vi "Create Data Channel.vi"(8 "error in (no error)":errorcluster, 9 "Channel":T1 {"Address" format="%.0x"}, 10 "Name":string, 11 "Parent Section":refnum<k24>) -> (0 "error out":errorcluster, 2 "New Data Channel":refnum<k24>, 3 "Parent Section Duplicate":refnum<k24>, 4 "Newly Created?":bool, 6 "Adds Warn?":bool caption="Address Within NIVS Reserved Range?")   [LabVIEW 2010, in "RefMem PtByPt System Definition API.lvlib"]
doc: "Create a data channel to contain the value at the specified reflective memory address."
uses:
  RefMem PtByPt System Definition API.lvlib
  Channel Config.ctl
  Custom Device/Controls/Data Channel Type.ctl
  NationalInstruments.VeriStand.SystemDefinitionAPI
  <vilib>/NI Veristand/Custom Device API/Custom Device Channel Type.ctl
  Custom Device/Controls/Global.vi
  Custom Device/RefMem PtByPt Custom Device.lvlib
  <vilib>/NI Veristand/Custom Device API/Custom Device API.lvlib
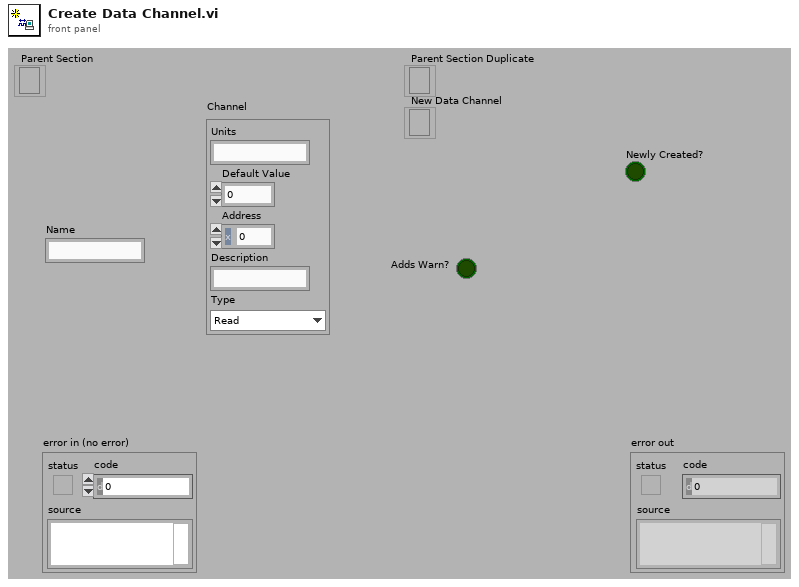
[diagram p1: front panel]
types:
  T1 = typedef "RefMem PtByPt System Definition API.lvlib/Channel Config.ctl" = cluster{"Units":string, "Default Value":dbl, "Address":u32, "Description":string, "Type":T2}
  T2 = typedef "RefMem PtByPt Custom Device.lvlib/Data Channel Type.ctl" = enum16{"Read", "Write"}
  T3 = typedef "Custom Device API.lvlib/Custom Device Channel Type.ctl" = enum16{"Input", "Output"}
  T4 = typedef "Custom Device API.lvlib/Custom Device Pointer.ctl" = refnum<k24>
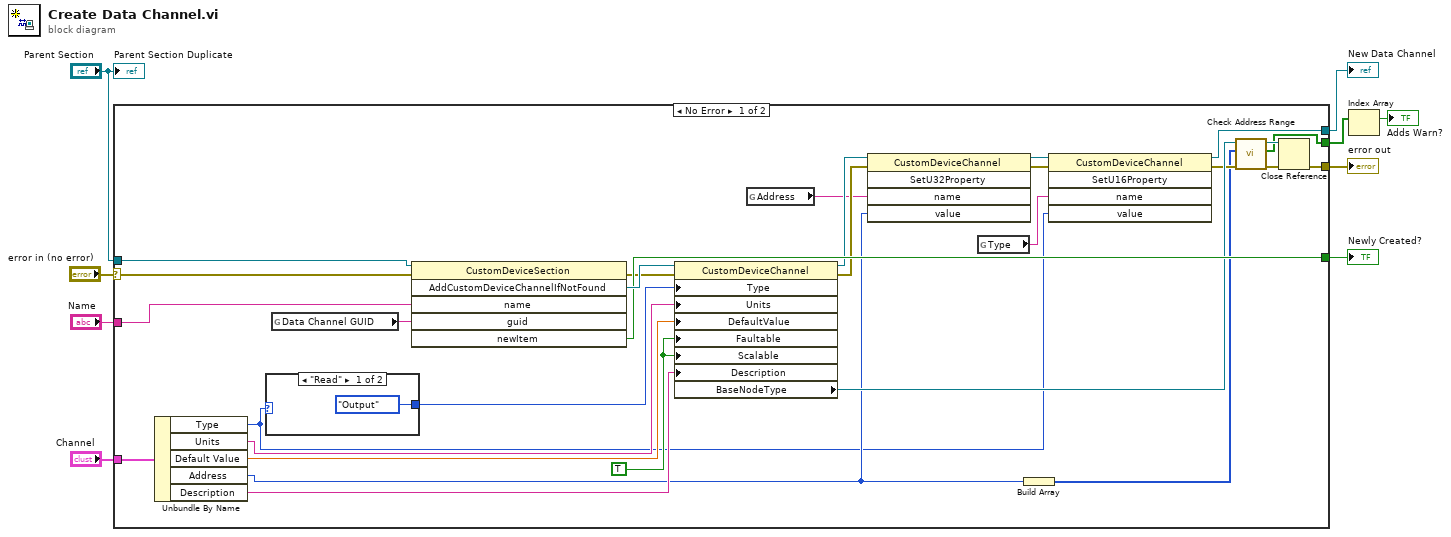
[diagram p0: block diagram]
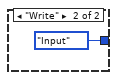
[diagram p2: hidden frame]
diagram:
  n1 = case shown="No Error" "error in (no error)" {
    selector: "error in (no error)" -> [w37 w41]
    tunnel: [w18 w41] -> w7
    tunnel: "Parent Section" -> [w38 _]
    tunnel: [w14 _] -> w3
    tunnel: [w35 _] -> w8
    tunnel: "Name" -> [w34 _]
    tunnel: "Channel" -> [w33 _]
    tunnel: [w20 _] -> w2
    frame No Error {
      w29 = TRUE ("Faultable")
      n2 = Unbundle By Name(w33) -> ("Type"=w11:T2, "Units"=w32:string, "Default Value"=w31:dbl, "Address"=w19:u32, "Description"=w24:string)
      n3 = case shown="\"Read\"" w11 {
        tunnel: [Custom_Device_Channel_Type."Output" ("Type") Custom_Device_Channel_Type."Input" ("Type")] -> w17
        frame "Read" {
        }
        frame "Write" {
        }
      }
      n4 = global read "Global.vi" "Data Channel GUID"() -> (w30:string)
      n5 = invoke class="CustomDeviceSection" method="AddCustomDeviceChannelIfNotFound"(reference=w38, error in=w37, "name"=w34, "guid"=w30) -> (error out=w28:errorcluster, "AddCustomDeviceChannelIfNotFound"=w36:refnum<k24>, "newItem"=w35:bool)  [unwired: 2 in, 3 out]
      n6 = property class="CustomDeviceChannel"(reference=w36, error in=w28, "Type"=w17, "Units"=w32, "DefaultValue"=w31, "Faultable"=w29, "Scalable"=w29, "Description"=w24) -> (reference out=w27:refnum<k24>, error out=w26:errorcluster, "BaseNodeType"=w23:refnum<k24>)
      n7 = global read "Global.vi" "Address"() -> (w25:string)
      n8 = invoke class="CustomDeviceChannel" method="SetU32Property"(reference=w27, error in=w26, "name"=w25, "value"=w19) -> (reference out=w16:refnum<k24>, error out=w15:errorcluster)  [unwired: 1 in, 3 out]
      n9 = global read "Global.vi" "Type"() -> (w12:string)
      n10 = Build Array(w19) -> (w10:u32[])
      n11 = invoke class="CustomDeviceChannel" method="SetU16Property"(reference=w16, error in=w15, "name"=w12, "value"=w11) -> (reference out=w14:refnum<k24>, error out=w13:errorcluster)  [unwired: 1 in, 3 out]
      n12 = call "Check Address Range.vi"("error in (no error)"=w13, "Addresses"=w10, "Node Pointer In"=w23) -> ("error out"=w22:errorcluster, "Inside NIVS Range"=w20:bool[], "Node Pointer dup"=w21:T4)  [unwired: 6 in]
      n13 = Close Reference(reference=w21, error in (no error)=w22) -> (error out=w18:errorcluster)
    }
    frame Error {
    }
  }
  "error out" <- w7
  "Newly Created?" <- w8
  "New Data Channel" <- w3
  n14 = Index Array(array=w2) -> (element=→"Adds Warn?":bool)  [unwired: 1 in]
  "Parent Section Duplicate" <- "Parent Section"
